vi "SQL_Server.vi"(8 "error in (no error)":errorcluster, 11 "Command Text":string) -> (0 "error out":errorcluster, 3 "status":bool)   [LabVIEW 2017]
panel:
  out "Data":string[][](array[string])
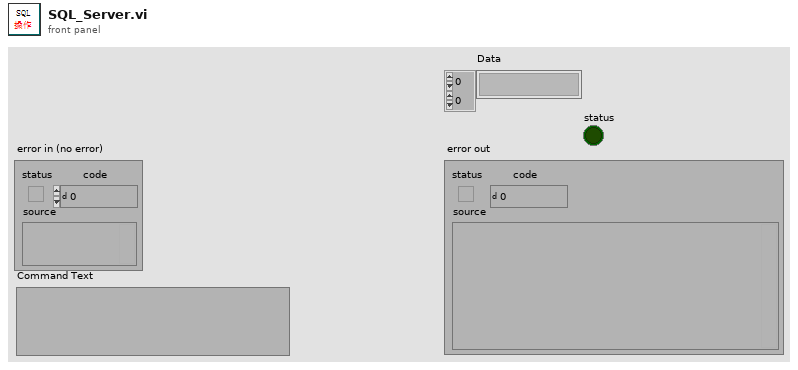
[diagram p1: front panel]
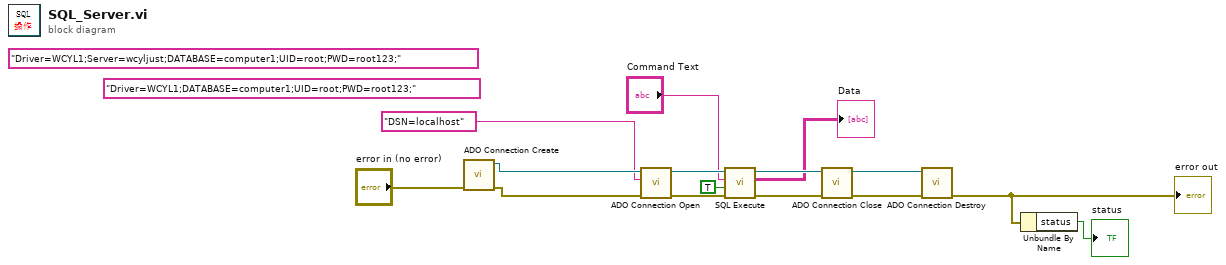
[diagram p0: block diagram]
diagram:
  (unwired) "Driver=WCYL1;DATABASE=computer1;UID=root;PWD=root123;" ("ConnectionString")
  (unwired) "Driver=WCYL1;Server=wcyljust;DATABASE=computer1;UID=root;PWD=root123;" ("ConnectionString")
  n1 = call <userlib>:"ADO Connection Create.vi"("error in (no error)"="error in (no error)") -> ("error out"=w13:errorcluster, "ADODB._Connection Out"=w14:refnum<k7>)  [unwired: 9 in]
  n2 = call <userlib>:"ADO Connection Open.vi"("error in (no error)"=w13, "ConnectionString"="DSN=localhost", "ADODB._Connection In"=w14) -> ("error out"=w11:errorcluster, "ADODB._Connection Out"=w12:refnum<k7>)  [unwired: 7 in]
  n3 = call <userlib>:"SQL Execute.vi"("error in (no error)"=w11, "Return Data (T)"=TRUE, "Command Text"="Command Text", "ADODB._Connection In"=w12) -> ("error out"=w7:errorcluster, "Data"=→"Data":string[][], "ADODB._Connection Out"=w8:refnum<k7>)  [unwired: 4 in, 1 out]
  n4 = call <userlib>:"ADO Connection Close.vi"("error in (no error)"=w7, "ADODB._Connection In"=w8) -> ("error out"=w5:errorcluster, "ADODB._Connection Out"=w6:refnum<k7>)  [unwired: 8 in]
  n5 = call <userlib>:"ADO Connection Destroy.vi"("error in (no error)"=w5, "ADODB._Connection In"=w6) -> ("error out"=w4:errorcluster)  [unwired: 9 in]
  "error out" <- w4
  n6 = Unbundle By Name(w4) -> ("status"=→"status":bool)
